vi "LIA Vrms2 to dBm Real.vi"(11 "Power Spectrum / PSD":cluster{"f0":dbl, "df":dbl, "magnitude":dbl[]}) -> (2 "output cluster":cluster{"f0":dbl, "df":dbl, "magnitude":dbl[]}, 3 "Power Spectrum / PSD (dBm)":cluster{"f0":dbl, "df":dbl, "magnitude":dbl[]})   [LabVIEW 2018]
uses:
  <vilib>/Analysis/baseanly.llb/Mean (DBL).vi
  <vilib>/Analysis/NI_AALBase.lvlib
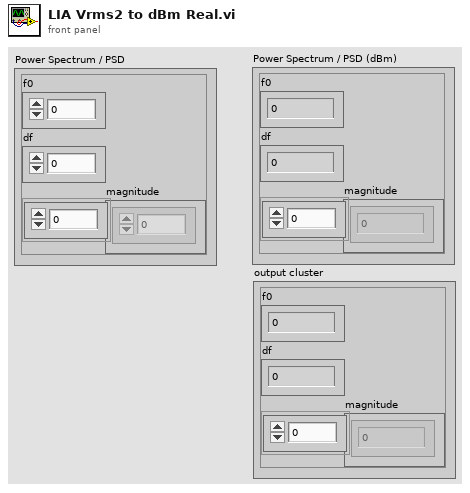
[diagram p1: front panel]
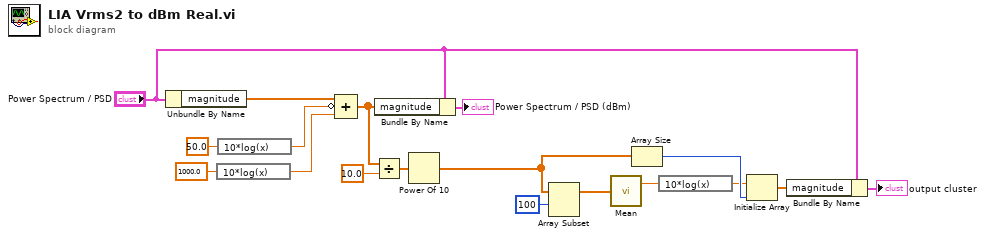
[diagram p0: block diagram]
diagram:
  n1 = Unbundle By Name("Power Spectrum / PSD") -> ("magnitude"=w17:dbl[])
  n2 = expression code="10*log(x)"(1000.0) -> (w13:dbl)
  n3 = expression code="10*log(x)"(50.0) -> (w16:dbl)
  n4 = Compound Arithmetic op=ADD(w17, invert w16, w13) -> (w12:dbl[])
  n5 = Divide(x=w12, y=10.0) -> (x/y=w11:dbl[])
  n6 = Bundle By Name(cluster="Power Spectrum / PSD", "magnitude"=w12) -> (→"Power Spectrum / PSD (dBm)":cluster{"f0":dbl, "df":dbl, "magnitude":dbl[]})
  n7 = Power Of 10(x=w11) -> (10^x=w7:dbl[])
  n8 = Array Subset(array=w7, index=100) -> (w2:dbl[])  [unwired: 1 in]
  n9 = call-poly <vilib>:"Mean.vi"("X"=w2) -> ("mean"=w9:dbl)  [unwired: 1 out]
  n10 = Array Size(array=w7) -> (size(s)=w6:i32)
  n11 = expression code="10*log(x)"(w9) -> (w5:dbl)
  n12 = Initialize Array(w5, w6) -> (w4:dbl[])
  n13 = Bundle By Name(cluster="Power Spectrum / PSD", "magnitude"=w4) -> (→"output cluster":cluster{"f0":dbl, "df":dbl, "magnitude":dbl[]})
